vi "Measure all.vi"(5 "Path loss compensation":bool=TRUE, 7 "PathControl in":refnum<class "PathControl.lvclass">, 8 "Error In":errorcluster, 9 "SG":i32, 10 "Frequency":dbl, 11 "Power Meter classes":refnum<class "Power Meter.lvclass">[](array[class])) -> (0 "Error Out":errorcluster, 1 "Power readings":dbl[](array[numeric]), 2 "Power results":T1[](array[typedef]), 3 "Power Meter classes":refnum<class "Power Meter.lvclass">[](array[class]), 4 "Calibration values":cluster{"Name":string, "Value":string}[](array[cluster]))   [LabVIEW 2020, in "Power Meter.lvclass"]
uses:
  Power Meter.lvclass
  Path Control/PathControl.lvclass
  XML Handler/Controls/Result Cluster.ctl
  Path Control/Paths.ctl
  XML Handler/XML Handler.lvclass
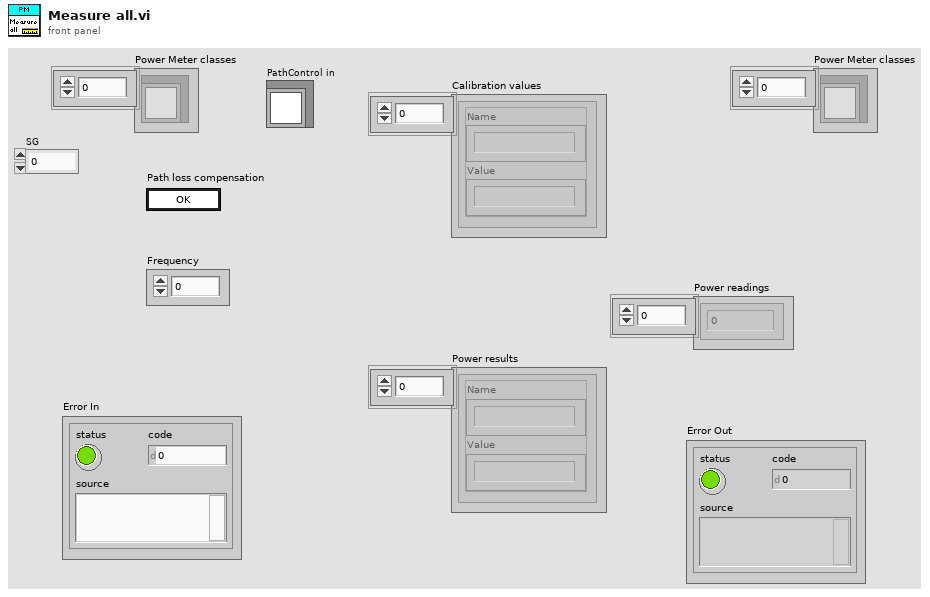
[diagram p1: front panel]
types:
  T1 = typedef "XML Handler.lvclass/Result Cluster.ctl" = cluster{"Name":string, "Value":string}
  T2 = typedef "PathControl.lvclass/Paths.ctl" = enum16{"SigGen 1 -> DUT", "SigGen 2 -> DUT", "SigGen 1 -> PM 1", "SigGen 1 -> PM 2", "DUT -> SA", "DUT -> PM 2", "VSG -> DUT", "SigGen 2 -> PM 1", "SigGen 2 -> PM 2"}
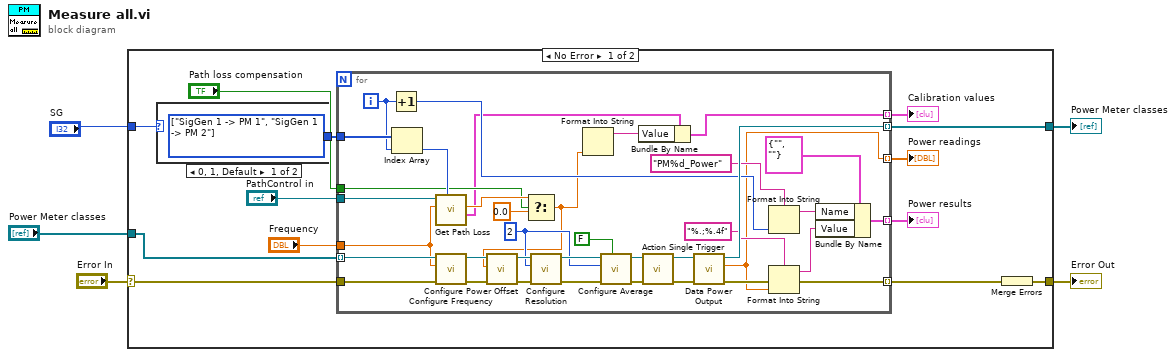
[diagram p0: block diagram]
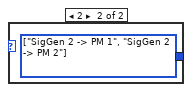
[diagram p2: hidden frame]
diagram:
  n1 = case shown="No Error" "Error In" {
    selector: "Error In" -> [w8 w58]
    tunnel: "Power Meter classes" -> [w12 w59]
    tunnel: [w11 w59] -> w4
    tunnel: [w9 w58] -> w3
    tunnel: "SG" -> [w6 _]
    frame No Error {
      n2 = case shown="0, 1, Default" w6 {
        tunnel: [w19 w20] -> w16
        frame 0, 1, Default {
          w19 = T2[] [enum."SigGen 1 -> PM 1", enum."SigGen 1 -> PM 2"] items=["SigGen 1 -> DUT", "SigGen 2 -> DUT", "SigGen 1 -> PM 1", "SigGen 1 -> PM 2", "DUT -> SA", "DUT -> PM 2", "VSG -> DUT", "SigGen 2 -> PM 1", "SigGen 2 -> PM 2"]
        }
        frame 2 {
          w20 = T2[] [enum."SigGen 2 -> PM 1", enum."SigGen 2 -> PM 2"] items=["SigGen 1 -> DUT", "SigGen 2 -> DUT", "SigGen 1 -> PM 1", "SigGen 1 -> PM 2", "DUT -> SA", "DUT -> PM 2", "VSG -> DUT", "SigGen 2 -> PM 1", "SigGen 2 -> PM 2"]
        }
      }
      n3 = for {
        tunnel: w12 -> [w53] mode=indexing
        tunnel: [w52] -> w11 mode=indexing
        tunnel: "Frequency" -> [w50]
        tunnel: [w45] -> w13 mode=indexing
        tunnel: "PathControl in" -> [w42]
        tunnel: w16 -> [w41]
        tunnel: [w23] -> w17 mode=indexing
        tunnel: w8 -> [w51]
        tunnel: [w37] -> w10 mode=indexing
        tunnel: [w28] -> w18 mode=indexing
        tunnel: "Path loss compensation" -> [w26]
        i -> [w39]
        w30 = 2 ("Resolution")
        n4 = Increment(x=w39) -> (x+1=w44:i32)
        n5 = Index Array(array=w41, index=w39) -> (element=w40:T2)
        n6 = call "Get Path Loss.vi"("Path"=w40, "Frequency [Hz]"=w50, "PathControl in"=w42) -> ("Parameter"=w24:cluster{"Name":string, "Value":string}, "Insertion Loss (dB)"=w27:dbl)  [unwired: 5 in, 2 out]
        n7 = call-dynamic "Configure Frequency.vi"("error in (no error)"=w51, "Frequency"=w50, "Power Meter in"=w53) -> ("error out"=w54:errorcluster, "Power Meter out"=w57:refnum<class "Power Meter.lvclass">)  [unwired: 7 in]
        n8 = Select(t=w27, s=w26, f=0.0) -> (s? t:f=w22:dbl)
        n9 = call-dynamic "Configure Power Offset.vi"("error in (no error)"=w54, "Power Offset"=w22, "Power Meter in"=w57) -> ("error out"=w35:errorcluster, "Power Meter out"=w36:refnum<class "Power Meter.lvclass">)  [unwired: 7 in]
        n10 = call-dynamic "Configure Resolution.vi"("error in (no error)"=w35, "Resolution"=w30, "Power Meter in"=w36) -> ("error out"=w33:errorcluster, "Power Meter out"=w34:refnum<class "Power Meter.lvclass">)  [unwired: 7 in]
        n11 = Format Into String(w22) -> (resulting string=w21:string)  [unwired: 3 in, 1 out]
        n12 = call-dynamic "Configure Average.vi"("Average on"=FALSE, "error in (no error)"=w33, "Average Count"=w30, "Power Meter in"=w34) -> ("error out"=w31:errorcluster, "Power Meter out"=w32:refnum<class "Power Meter.lvclass">)  [unwired: 6 in]
        n13 = Bundle By Name(cluster=w24, "Value"=w21) -> (w23:cluster{"Name":string, "Value":string})
        n14 = call-dynamic "Action Single Trigger.vi"("error in (no error)"=w31, "Power Meter in"=w32) -> ("error out"=w56:errorcluster, "Power Meter out"=w55:refnum<class "Power Meter.lvclass">)  [unwired: 8 in]
        n15 = call-dynamic "Data Power Output.vi"("error in (no error)"=w56, "Power Meter in"=w55) -> ("error out"=w38:errorcluster, "Power Out"=w28:dbl, "Power Meter out"=w52:refnum<class "Power Meter.lvclass">)  [unwired: 7 in]
        n16 = Format Into String(format string="PM%d_Power", w44) -> (resulting string=w47:string)  [unwired: 2 in, 1 out]
        n17 = Format Into String(format string="%.;%.4f", error in=w38, w28) -> (resulting string=w49:string, error out=w37:errorcluster)  [unwired: 1 in]
        n18 = Bundle By Name(cluster=T1 {"Name"="", "Value"=""} ("new element/subarray"), "Name"=w47, "Value"=w49) -> (w45:T1)
      }
      "Power readings" <- w18
      "Calibration values" <- w17
      "Power results" <- w13
      n19 = Merge Errors(w10) -> (w9:errorcluster)
    }
    frame Error {
    }
  }
  "Power Meter classes" <- w4
  "Error Out" <- w3
